vi "Get Attribute U32.vi"(8 "error in":errorcluster, 10 "Attribute":string, 11 "Config from JSON in":refnum<class "Config from JSON.lvclass">) -> (0 "error out":errorcluster, 2 "Value":u32, 3 "Config from JSON out":refnum<class "Config from JSON.lvclass">)   [LabVIEW 2024, in "Config from JSON.lvclass"]
uses:
  Config from JSON.lvclass
  Config from JSON.lvclass/Config from JSON.ctl
  <vilib>/JDP Science/JSONtext/LVClass Serializer/JSONtext LVClass Serializer.lvclass
  a3157557-e90b-440c-9c78-9e22d97c805f.vi
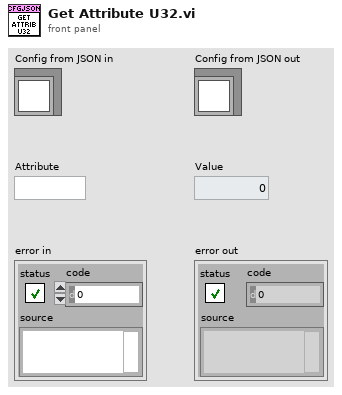
[diagram p1: front panel]
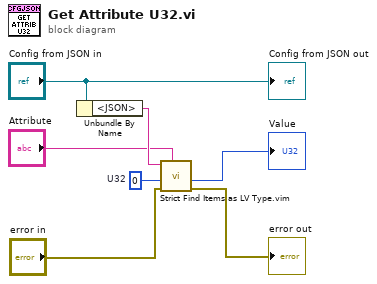
[diagram p0: block diagram]
diagram:
  w3 = u32 0  # U32
  n1 = Unbundle By Name("Config from JSON in") -> ("<JSON>"=w6:string)
  n2 = call "Strict Find Items as LV Type.vim"("$Path or Item Name"="Attribute", "error in"="error in", "Data Type and Default Value"=w3, "<JSON>"=w6) -> ("error out"=→"error out":errorcluster, "Data out"=→"Value":u32)  [unwired: 5 in, 1 out]
  "Config from JSON out" <- "Config from JSON in"
